vi "Hide.vi"(0 "LV MDI in":refnum<class "LV MDI.lvclass">, 5 "Doc UID[]":string[](array[string]), 11 "error in (no error)":errorcluster) -> (4 "LV MDI out":refnum<class "LV MDI.lvclass">, 15 "error out":errorcluster)   [LabVIEW 2019, in "LV MDI.lvclass"]
doc: "Hide the document in container."
uses:
  LV MDI.lvclass
  Document/Document base/Document.lvclass/Document.ctl
  Document/Document base/property/Read Doc Hwnd.vi
  Document/Document base/Document.lvclass
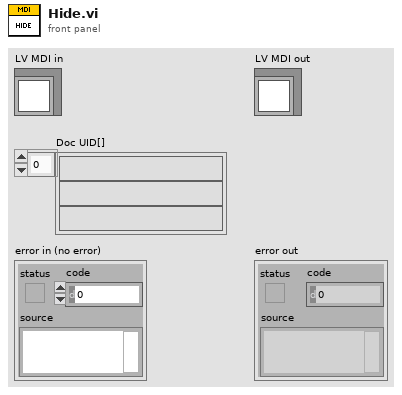
[diagram p1: front panel]
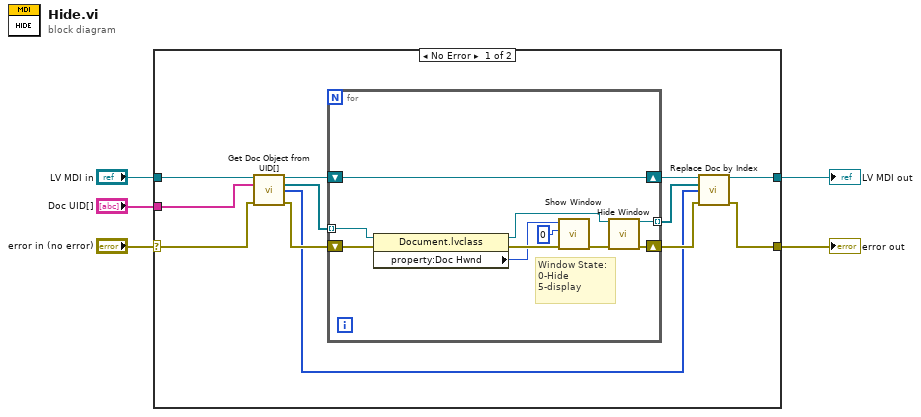
[diagram p0: block diagram]
diagram:
  n1 = case shown="No Error" "error in (no error)" {
    selector: "error in (no error)" -> [w13 w29]
    tunnel: [w8 w29] -> w4
    tunnel: [w10 w28] -> w2
    tunnel: "LV MDI in" -> [w14 w28]
    tunnel: "Doc UID[]" -> [w12 _]
    frame No Error {
      n2 = call "Get Doc Object from UID[].vi"("LV MDI"=w14, "Doc ÙID[]"=w12, "error in"=w13) -> ("LV MDI"=w15:refnum<class "LV MDI.lvclass">, "Doc obj[]"=w16:refnum<class "Document.lvclass">[], "Doc index[]"=w7:i32[], "error Out"=w17:errorcluster)  [unwired: 9 in]
      n3 = for {
        shift-right: [w25] -> w9
        shift-left: w17 -> [w26]
        tunnel: w16 -> [w27] mode=indexing
        shift-right: [w22] -> w11
        shift-left: w15 -> [w22]
        tunnel: [w23] -> w6 mode=indexing
        # "Window State:\n0-Hide\n5-display"
        n4 = property class="Document.lvclass"(reference=w27, error in=w26) -> (reference out=w24:refnum<class "Document.lvclass">, error out=w21:errorcluster, "property:Doc Hwnd"=w18:u32)
        n5 = call "Show Window.vi"("error in (no error)"=w21, "Window State"=u32 0, "hwnd"=w18) -> ("error out"=w20:errorcluster)  [unwired: 7 in, 1 out]
        n6 = call-dynamic "Hide Window.vi"("Document in"=w24, "error in (no error)"=w20) -> ("Document out"=w23:refnum<class "Document.lvclass">, "error out"=w25:errorcluster)  [unwired: 12 in]
      }
      n7 = call "Replace Doc by Index.vi"("LV MDI in"=w11, "Doc Class Object[]"=w6, "Doc index[]"=w7, "error in (no error)"=w9) -> ("LV MDI out"=w10:refnum<class "LV MDI.lvclass">, "error out"=w8:errorcluster)  [unwired: 10 in]
    }
    frame Error {
    }
  }
  "error out" <- w4
  "LV MDI out" <- w2
